vi "Queue Driver.vi"(0 "queue name":string, 5 "state and data":T1, 7 "array of state and data":T1[](array[typedef]), 11 "error in":errorcluster, 13 "queue operation":T2) -> (4 "dequeued state":string, 6 "dequeued data":variant, 15 "error out":errorcluster)   [LabVIEW 2021, in "Game of Life.lvlib" / "Queue Driver.lvlib"]
uses:
  Queue Driver.lvlib
  Queue Operations.ctl
  Queue State and Data.ctl
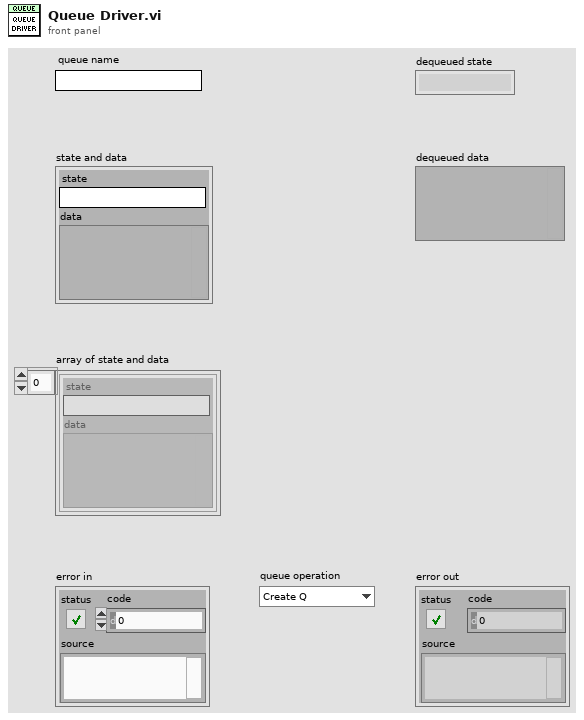
[diagram p1: front panel]
types:
  T1 = typedef "Game of Life.lvlib/Queue Driver.lvlib/Queue State and Data.ctl" = cluster{"state":string, "data":variant}
  T2 = typedef "Game of Life.lvlib/Queue Driver.lvlib/Queue Operations.ctl" = enum16{"Create Q", "Enqueue", "Enqueue N", "Enstack", "Enstack N", "Dequeue", "Flush", "Release"}
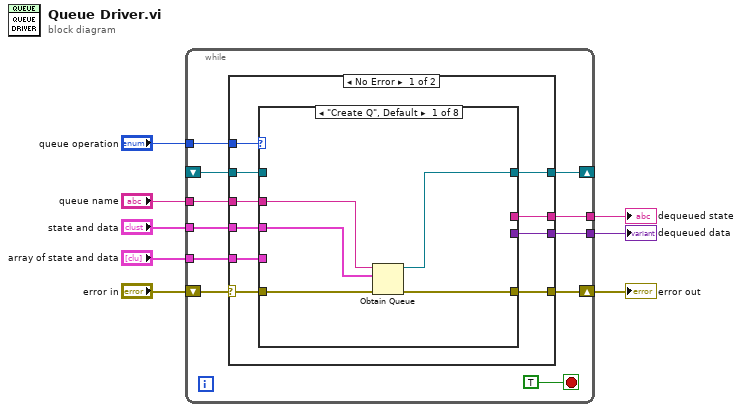
[diagram p0: block diagram]
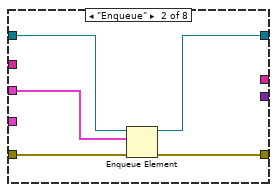
[diagram p2: hidden frame]
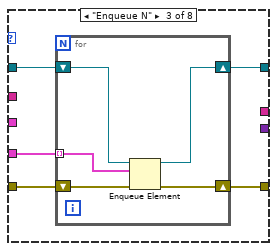
[diagram p3: hidden frame]
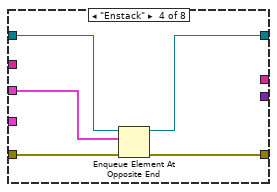
[diagram p4: hidden frame]
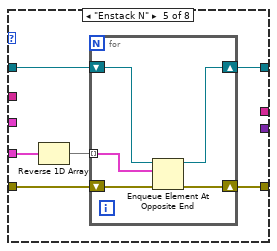
[diagram p5: hidden frame]
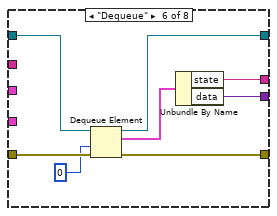
[diagram p6: hidden frame]
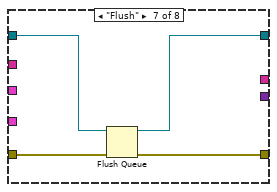
[diagram p7: hidden frame]
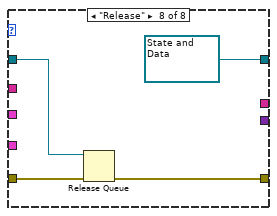
[diagram p8: hidden frame]
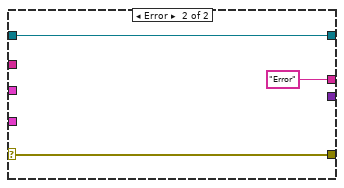
[diagram p9: hidden frame]
diagram:
  n1 = while {
    tunnel: "queue operation" -> [w19]
    tunnel: "queue name" -> [w18]
    shift-right: [w15] -> _
    shift-left: _ -> [w14]
    tunnel: "state and data" -> [w17]
    tunnel: "array of state and data" -> [w16]
    shift-right: [w13] -> w3
    shift-left: "error in" -> [w12]
    tunnel: [w10] -> w2
    tunnel: [w9] -> w1
    stop <- TRUE stop-if-true
    n2 = case shown="No Error" w12 {
      selector: w12 -> [w21 w83]
      tunnel: w19 -> [w29 _]
      tunnel: w18 -> [w28 _]
      tunnel: w17 -> [w27 _]
      tunnel: w16 -> [w20 _]
      tunnel: [w26 w84] -> w15
      tunnel: w14 -> [w25 w84]
      tunnel: [w24 w83] -> w13
      tunnel: [w23 "Error" ("State")] -> w10
      tunnel: [w22 _] -> w9
      frame No Error {
        n3 = case shown="\"Create Q\", Default" w29 {
          tunnel: w28 -> [w34 _ _ _ _ _ _ _]
          tunnel: w27 -> [w33 w38 _ w52 _ _ _ _]
          tunnel: w20 -> [_ _ w44 _ w56 _ _ _]
          tunnel: [w32 w37 w42 w53 w59 w70 w76 refnum<queue> refnum ("queue out")] -> w26
          tunnel: w25 -> [_ w39 w43 w54 w60 w67 w77 w81]
          tunnel: [w30 w35 w40 w50 w57 w69 w74 w78] -> w24
          tunnel: w21 -> [w31 w36 w41 w51 w58 w68 w75 w79]
          tunnel: [_ _ _ _ _ w72 _ _] -> w23
          tunnel: [_ _ _ _ _ w71 _ _] -> w22
          frame "Create Q", Default {
            n4 = Obtain Queue(name (unnamed)=w34, element data type=w33, error in (no error)=w31) -> (queue out=w32:refnum<queue>, error out=w30:errorcluster)  [unwired: 2 in, 1 out]
          }
          frame "Enqueue" {
            n5 = Enqueue Element(queue=w39, element=w38, error in (no error)=w36) -> (queue out=w37:refnum<queue>, error out=w35:errorcluster)  [unwired: 1 in, 1 out]
          }
          frame "Enqueue N" {
            n6 = for {
              tunnel: w44 -> [w47] mode=indexing
              shift-right: [w48] -> w42
              shift-left: w43 -> [w49]
              shift-right: [w45] -> w40
              shift-left: w41 -> [w46]
              n7 = Enqueue Element(queue=w49, element=w47, error in (no error)=w46) -> (queue out=w48:refnum<queue>, error out=w45:errorcluster)  [unwired: 1 in, 1 out]
            }
          }
          frame "Enstack" {
            n8 = Enqueue Element At Opposite End(queue=w54, element=w52, error in (no error)=w51) -> (queue out=w53:refnum<queue>, error out=w50:errorcluster)  [unwired: 1 in, 1 out]
          }
          frame "Enstack N" {
            n9 = Reverse 1D Array(array=w56) -> (reversed array=w55:T1[])
            n10 = for {
              shift-right: [w64] -> w59
              shift-left: w60 -> [w65]
              shift-right: [w62] -> w57
              shift-left: w58 -> [w63]
              tunnel: w55 -> [w61] mode=indexing
              n11 = Enqueue Element At Opposite End(queue=w65, element=w61, error in (no error)=w63) -> (queue out=w64:refnum<queue>, error out=w62:errorcluster)  [unwired: 1 in, 1 out]
            }
          }
          frame "Dequeue" {
            n12 = Dequeue Element(queue=w67, timeout in ms (-1)=0, error in (no error)=w68) -> (queue out=w70:refnum<queue>, element=w73:T1, error out=w69:errorcluster)  [unwired: 1 out]
            n13 = Unbundle By Name(w73) -> ("state"=w72:string, "data"=w71:variant)
          }
          frame "Flush" {
            n14 = Flush Queue(queue=w77, error in (no error)=w75) -> (queue out=w76:refnum<queue>, error out=w74:errorcluster)  [unwired: 1 out]
          }
          frame "Release" {
            n15 = Release Queue(queue=w81, error in (no error)=w79) -> (error out=w78:errorcluster)  [unwired: 1 in, 2 out]
          }
        }
      }
      frame Error {
      }
    }
  }
  "error out" <- w3
  "dequeued state" <- w2
  "dequeued data" <- w1
